vi "SSL Detection Robots Delete Invalids.vi"(5 "Now":timestamp, 7 "Life Time":dbl=1.0, 11 "Robots In":T1[](array[typedef]) {"height" format="%+4.3f"; "pixel_y" format="%+4.3f"; "pixel_x" format="%+4.3f"; "orientation" format="%+4.3f"; "y" format="%+4.3f"; "confidence" format="%4.3f"; "x" format="%+4.3f"}) -> (3 "Robots Out":T1[](array[typedef]) {"height" format="%+4.3f"; "pixel_y" format="%+4.3f"; "pixel_x" format="%+4.3f"; "orientation" format="%+4.3f"; "y" format="%+4.3f"; "confidence" format="%4.3f"; "x" format="%+4.3f"})   [LabVIEW 2016]
uses:
  SSL Detection Robot.ctl
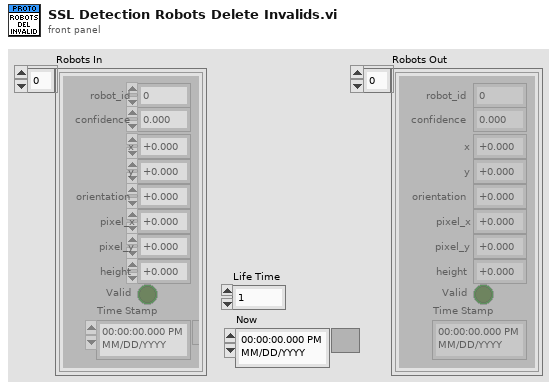
[diagram p1: front panel]
types:
  T1 = typedef "SSL Detection Robot.ctl" = cluster{"x":sgl, "robot_id":u32, "confidence":sgl, "y":sgl, "orientation":sgl, "pixel_x":sgl, "pixel_y":sgl, "height":sgl, "Valid":bool, "Time Stamp":timestamp}
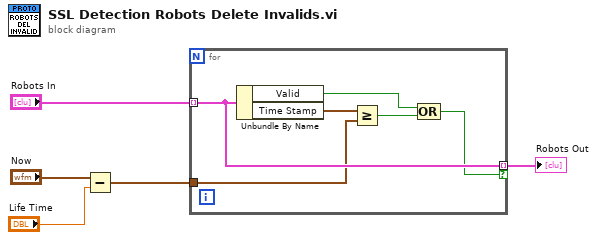
[diagram p0: block diagram]
diagram:
  n1 = Subtract(x="Now", y="Life Time") -> (x-y=w1:timestamp)
  n2 = for {
    tunnel: "Robots In" -> [w11] mode=indexing
    tunnel: [w11] -> w4 mode=indexing if=w10
    tunnel: w1 -> [w8]
    n3 = Unbundle By Name(w11) -> ("Valid"=w7:bool, "Time Stamp"=w9:timestamp)
    n4 = Greater Or Equal?(x=w9, y=w8) -> (x >= y?=w6:bool)
    n5 = Compound Arithmetic op=OR(w7, w6) -> (w10:bool)
  }
  "Robots Out" <- w4
